vi "Build XY Waveform.vi"(10 "New Temps":dbl[](array[numeric]), 11 "Waveforms in":waveform(dbl)[](array[waveform])) -> (3 "Waveforms out":waveform(dbl)[](array[waveform]))   [LabVIEW 2021]
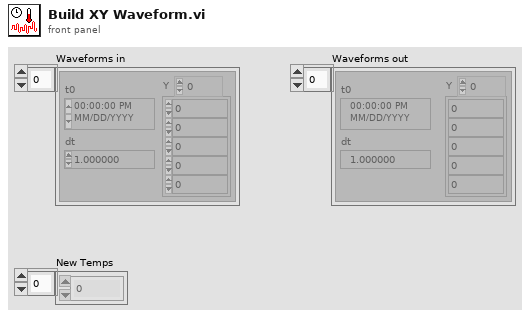
[diagram p1: front panel]
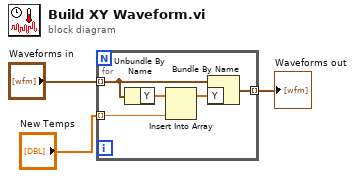
[diagram p0: block diagram]
diagram:
  n1 = for {
    tunnel: "Waveforms in" -> [w5] mode=indexing
    tunnel: "New Temps" -> [w7] mode=indexing
    tunnel: [w4] -> w2 mode=indexing
    n2 = Unbundle By Name(w5) -> ("Y"=w8:dbl[])
    n3 = Insert Into Array(array=w8, new element=w7) -> (w6:dbl[])  [unwired: 1 in]
    n4 = Bundle By Name(cluster=w5, "Y"=w6) -> (w4:waveform(dbl))
  }
  "Waveforms out" <- w2
